vi "Work.vi"(8 "error in (no error)":errorcluster, 9 "Outputs":refnum<class "Output.lvclass">[](array[class]), 10 "Inputs":refnum<class "Input.lvclass">[](array[class]), 11 "TestBlock in":refnum<class "TestBlock.lvclass">) -> (0 "error out":errorcluster, 3 "TestBlock out":refnum<class "TestBlock.lvclass">)   [LabVIEW 2020, in "TestBlock.lvclass"]
uses:
  TestBlock.lvclass
  Parallel Block/Input/Input.lvclass
  Parallel Block/Output/Output.lvclass
  TestBlock.lvclass/TestBlock.ctl
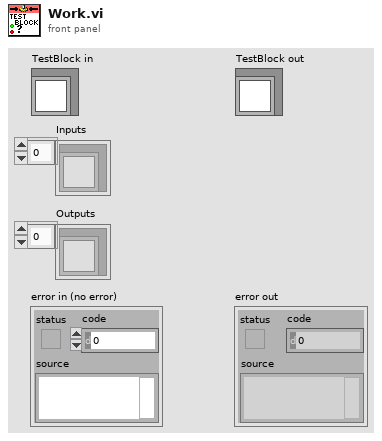
[diagram p1: front panel]
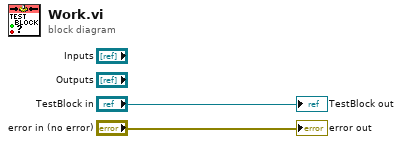
[diagram p0: block diagram]
diagram:
  "error out" <- "error in (no error)"
  "TestBlock out" <- "TestBlock in"
